vi "Upgrade Hardware ConfigurationI.vi"(8 "error in (no error)":errorcluster, 11 "Path":path) -> (0 "error out":errorcluster, 3 "name":string)   [LabVIEW 2023]
uses:
  Resources/Type Defs/Shutter Configuration.ctl
  Resources/Type Defs/Stage Configuration.ctl
  Resources/Type Defs/Microscope Configuration.ctl
  Resources/Type Defs/Camera Type.ctl
  Resources/Type Defs/Virtual Camera Configuration.ctl
  Resources/Type Defs/Laser Configuration.ctl
  Resources/Type Defs/Physical Camera Assignment.ctl
  Resources/Type Defs/Hardware Configuration.ctl
  Resources/Type Defs/Microscope Type.ctl
  Resources/Type Defs/DAQ Configuration.ctl
  <vilib>/Utility/xml.llb/Read From XML File(string).vi
  <vilib>/Utility/xml.llb/Write to XML File(string).vi
panel:
  # "Select a file to convert. It will be overwritten with the new version."
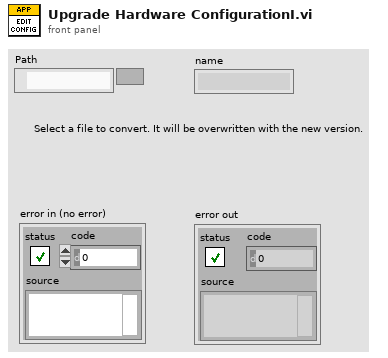
[diagram p1: front panel]
types:
  T1 = typedef "Microscope Type.ctl" = enum16{"Disable", "TE2000", "Eclipse Ti", "Ti2"}
  T2 = typedef "Camera Type.ctl" = enum16{"Hamamatsu", "Andor", "Photometrics"}
  T3 = cluster{"Shutters":cluster{"IO Line":tag, "Name":string, "Wavelength":u16, "Max rate (Hz)":dbl}[], "Stage Configuration":cluster{"Serial Port":refnum<visa-resource-name>, "Forward Step (mm)":dbl, "Lane Length (mm)":dbl, "Lane Separation (mm)":dbl, "Stage Type":enum16{"Disabled", "ESP301", "Ti2", "Ludl", "ASI"}, "Autofocus Steps":i32, "Autofocus Range (um)":dbl, "Stage Limits":cluster{"Y Min":dbl, "Y Max":dbl, "X Min":dbl, "X Max":dbl}, "Slide (mm)":cluster{"top":dbl, "right":dbl, "width":dbl, "height":dbl}}, "Microscope Configuration":cluster{"Serial Port":refnum<visa-resource-name>, "Microscope Type":T1, "Detection Settings":cluster{"Name":string, "Filter Position":u16, "Optical Path":u16}[]}, "Virtual Camera Configuration":cluster{"Camera Type":T2, "Sync Line":tag}, "Laser Configuration":cluster{"Serial Port":refnum<visa-resource-name>, "Laser Type":enum16{"Disable", "Laser Quantum", "Coherent OBIS", "PRM1-Z8", "Coherent HOPS"}, "Polarizer Amplitude":dbl, "Polarizer Theta Zero":dbl, "Wavelength":u16}[], "Fluidics Configuration":cluster{"fluidics trigger line":tag}, "Installed Cameras":cluster{"Channel Name":string, "Serial Number":string, "Flip Vertically":bool, "Flip Horizontally":bool, "wavelength":i16, "photonsPerCount":dbl[]}[], "Power Meter Configuration":cluster{"Power Meter Type":enum16{"Disabled", "Thorlabs", "Newport", "Coherent"}, "attenuation":dbl, "instrument handle":refnum<visa-resource-name>}}
  T4 = typedef "Hardware Configuration.ctl" = cluster{"Stage Configuration":T5, "Microscope Configuration":T6, "Virtual Camera Configuration":T7, "Laser Configuration":T8[], "Installed Cameras":T9[], "Power Meter Configuration":cluster{"Power Meter Type":enum16{"Disabled", "Thorlabs", "Newport", "Coherent"}, "attenuation":dbl, "instrument handle":refnum<visa-resource-name>}, "DAQ Configuration":T10}
  T5 = typedef "Stage Configuration.ctl" = cluster{"Serial Port":refnum<visa-resource-name>, "Forward Step (mm)":dbl, "Lane Length (mm)":dbl, "Lane Separation (mm)":dbl, "Stage Type":enum16{"Disabled", "ESP301", "Ti2", "Ludl", "ASI"}, "Autofocus Steps":i32, "Autofocus Range (um)":dbl, "Stage Limits":cluster{"Y Min":dbl, "Y Max":dbl, "X Min":dbl, "X Max":dbl}, "Slide (mm)":cluster{"top":dbl, "right":dbl, "width":dbl, "height":dbl}}
  T6 = typedef "Microscope Configuration.ctl" = cluster{"Serial Port":refnum<visa-resource-name>, "Microscope Type":T1, "Detection Settings":cluster{"Name":string, "Filter Position":u16, "Optical Path":u16}[]}
  T7 = typedef "Virtual Camera Configuration.ctl" = cluster{"Camera Type":T2}
  T8 = typedef "Laser Configuration.ctl" = cluster{"Serial Port":refnum<visa-resource-name>, "Laser Type":enum16{"Disable", "Laser Quantum", "Coherent OBIS", "PRM1-Z8", "Coherent HOPS"}, "Polarizer Amplitude":dbl, "Polarizer Theta Zero":dbl, "Wavelength":u16}
  T9 = typedef "Physical Camera Assignment.ctl" = cluster{"Channel Name":string, "Serial Number":string, "Flip Vertically":bool, "Flip Horizontally":bool, "wavelength":i16, "photonsPerCount":dbl[]}
  T10 = typedef "DAQ Configuration.ctl" = cluster{"Shutters":T11[], "fluidics trigger line":tag, "camera trigger line":tag, "COM Port":refnum<visa-resource-name>}
  T11 = typedef "Shutter Configuration.ctl" = cluster{"IO Line":tag, "Name":string, "Wavelength":u16, "Max rate (Hz)":dbl}
  T12 = cluster{"Serial Port":refnum<visa-resource-name>, "Forward Step (mm)":dbl, "Lane Length (mm)":dbl, "Lane Separation (mm)":dbl, "Stage Type":enum16{"Disabled", "ESP301", "Ti2", "Ludl", "ASI"}, "Autofocus Steps":i32, "Autofocus Range (um)":dbl, "Stage Limits":cluster{"Y Min":dbl, "Y Max":dbl, "X Min":dbl, "X Max":dbl}, "Slide (mm)":cluster{"top":dbl, "right":dbl, "width":dbl, "height":dbl}}
  T13 = cluster{"Serial Port":refnum<visa-resource-name>, "Microscope Type":T1, "Detection Settings":cluster{"Name":string, "Filter Position":u16, "Optical Path":u16}[]}
  T14 = cluster{"Serial Port":refnum<visa-resource-name>, "Laser Type":enum16{"Disable", "Laser Quantum", "Coherent OBIS", "PRM1-Z8", "Coherent HOPS"}, "Polarizer Amplitude":dbl, "Polarizer Theta Zero":dbl, "Wavelength":u16}[]
  T15 = cluster{"Channel Name":string, "Serial Number":string, "Flip Vertically":bool, "Flip Horizontally":bool, "wavelength":i16, "photonsPerCount":dbl[]}[]
  T16 = cluster{"Power Meter Type":enum16{"Disabled", "Thorlabs", "Newport", "Coherent"}, "attenuation":dbl, "instrument handle":refnum<visa-resource-name>}
  T17 = cluster{"IO Line":tag, "Name":string, "Wavelength":u16, "Max rate (Hz)":dbl}[]
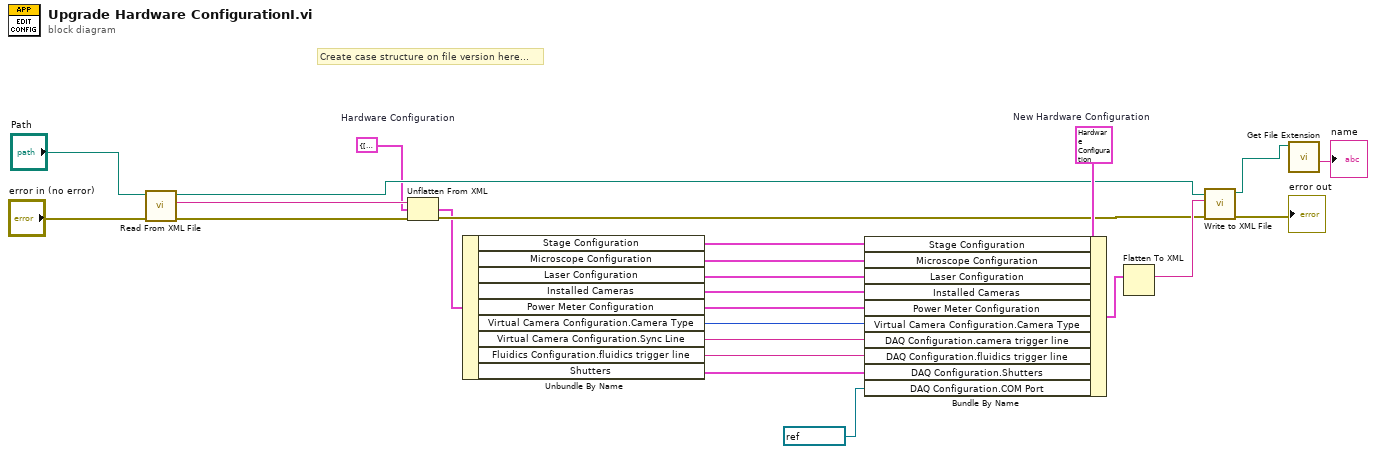
[diagram p0: block diagram]
diagram:
  w5 = T3 {"Shutters"=[], "Stage Configuration"={"Serial Port"="COM3", "Forward Step (mm)"=0.4, "Lane Length (mm)"=6.0, "Lane Separation (mm)"=0.8, "Stage Type"=enum."ESP301", "Autofocus Steps"=9, "Autofocus Range (um)"=30.0, "Stage Limits"={"Y Min"=-4.5, "Y Max"=3.0, "X Min"=-19.0, "X Max"=33.5}, "Slide (mm)"={"top"=-22300.0, "right"=-13000.0, "width"=60000.0, "height"=25400.0}}, "Microscope Configuration"={"Serial Port"="COM2", "Microscope Type"=enum."TE2000", "Detection Settings"=[]}, "Virtual Camera Configuration"={"Camera Type"=enum."Hamamatsu", "Sync Line"=""}, "Laser Configuration"=[], "Fluidics Configuration"={"fluidics trigger line"="Dev1/port2/line6"}, "Installed Cameras"=[], "Power Meter Configuration"={"Power Meter Type"=enum."Disabled", "attenuation"=53.2, "instrument handle"="USB0::0x1313::0x8075::P5001392::INSTR"}}  # Hardware Configuration
  w18 = T4 {"Stage Configuration"={"Serial Port"="COM3", "Forward Step (mm)"=0.4, "Lane Length (mm)"=6.0, "Lane Separation (mm)"=0.8, "Stage Type"=enum."ESP301", "Autofocus Steps"=9, "Autofocus Range (um)"=30.0, "Stage Limits"={"Y Min"=-4.5, "Y Max"=3.0, "X Min"=-19.0, "X Max"=33.5}, "Slide (mm)"={"top"=-22300.0, "right"=-13000.0, "width"=60000.0, "height"=25400.0}}, "Microscope Configuration"={"Serial Port"="COM2", "Microscope Type"=enum."TE2000", "Detection Settings"=[]}, "Virtual Camera Configuration"={"Camera Type"=enum."Hamamatsu"}, "Laser Configuration"=[], "Installed Cameras"=[], "Power Meter Configuration"={"Power Meter Type"=enum."Disabled", "attenuation"=53.2, "instrument handle"="USB0::0x1313::0x8075::P5001392::INSTR"}, "DAQ Configuration"={"Shutters"=[], "fluidics trigger line"="Dev1/port1/line1", "camera trigger line"="", "COM Port"="COM3"}}  # New Hardware Configuration
  # "Create case structure on file version here..."
  n1 = call-poly <vilib>:"Read From XML File.vi"("error in (no error)"="error in (no error)", "XML File Path"="Path") -> ("error out"=w15:errorcluster, "XML Elements"=w16:string, "XML File Path(duplicate)"=w13:path)  [unwired: 7 in]
  n2 = Unflatten From XML(xml string=w16, type=w5, error in (no error)=w15) -> (value=w9:T3, error out=w14:errorcluster)
  n3 = Unbundle By Name(w9) -> ("Stage Configuration"=w8:T12, "Microscope Configuration"=w7:T13, "Laser Configuration"=w10:T14, "Installed Cameras"=w11:T15, "Power Meter Configuration"=w12:T16, "Virtual Camera Configuration.Camera Type"=w4:T2, "Virtual Camera Configuration.Sync Line"=w3:tag, "Fluidics Configuration.fluidics trigger line"=w2:tag, "Shutters"=w1:T17)
  n4 = Bundle By Name(cluster=w18, "Stage Configuration"=w8, "Microscope Configuration"=w7, "Laser Configuration"=w10, "Installed Cameras"=w11, "Power Meter Configuration"=w12, "Virtual Camera Configuration.Camera Type"=w4, "DAQ Configuration.camera trigger line"=w3, "DAQ Configuration.fluidics trigger line"=w2, "DAQ Configuration.Shutters"=w1, "DAQ Configuration.COM Port"=refnum<visa-resource-name> "COM3") -> (w17:T4)
  n5 = Flatten To XML(6:w17) -> (2:w19:string)
  n6 = call-poly <vilib>:"Write to XML File.vi"("error in (no error)"=w14, "XML Input"=w19, "XML File Path"=w13) -> ("error out"=→"error out":errorcluster, "XML File Path(duplicate)"=w21:path)  [unwired: 6 in, 1 out]
  n7 = call <vilib>:"Get File Extension.vi"("file"=w21) -> ("filename without extension"=→"name":string)  [unwired: 6 in, 4 out]
